vi "test_decodeTxGenConfig.vi"() -> ()   [LabVIEW 2020]
uses:
  Shared/hardware_channels_tx.ctl
  Shared/channel_settings_tx.ctl
  Shared/Frame Payload Parameters.ctl
  Shared/Encoding (Arinc664).ctl
  Shared/RawFrame_entry.ctl
  <instrlib>/AIM GmbH/_AIM 664/_controls/queue_header_generic.ctl
  <instrlib>/AIM GmbH/_AIM 664/AIM664LV.lvlib
panel:
  out "tx gen config":T1 {"channel settings"."Payload Parameter Array"."Parameters"."encoding" items=["BNR", "BCD", "Discrete"]}
  out "last mod":timestamp
  out "error out":errorcluster
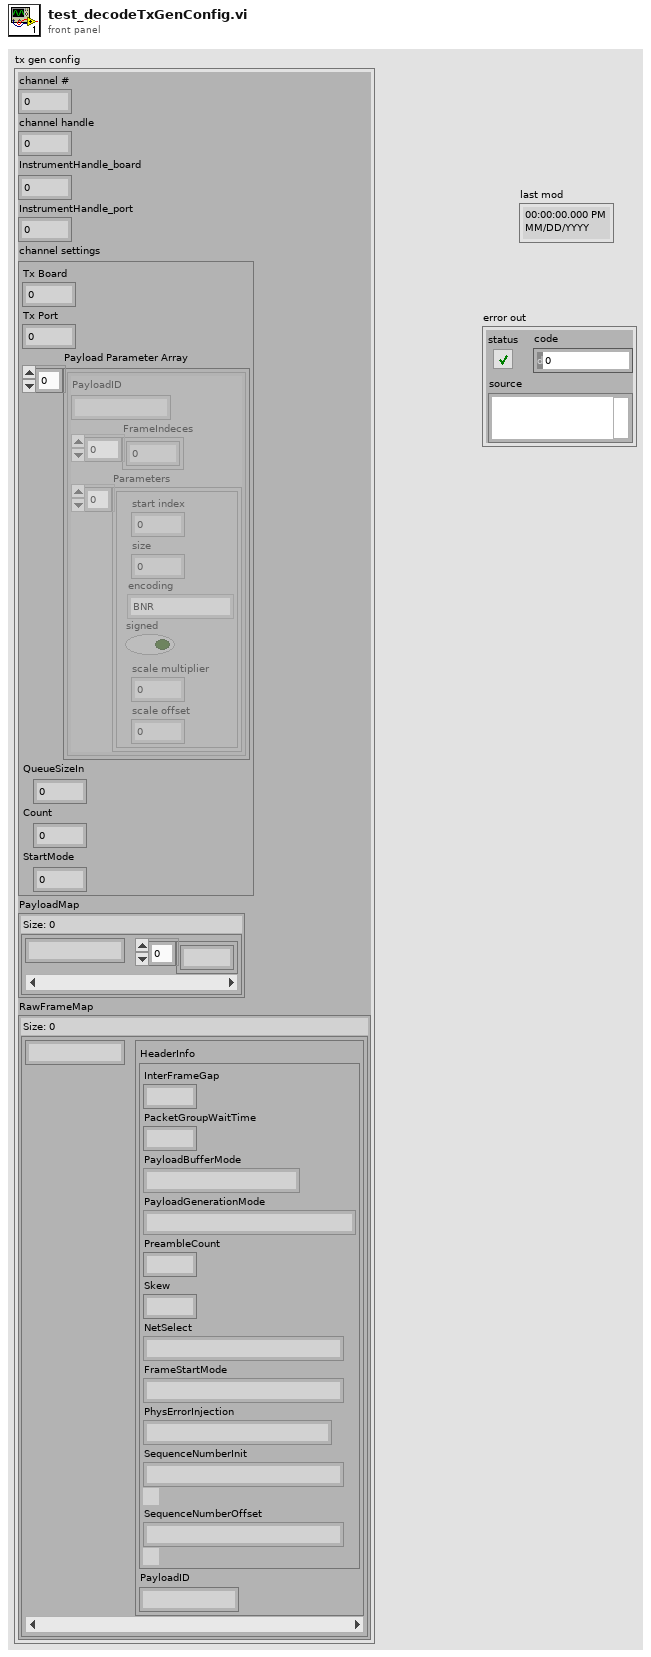
[diagram p1: front panel]
types:
  T1 = typedef "hardware_channels_tx.ctl" = cluster{"channel #":u16, "channel handle":u64, "InstrumentHandle_board":u32, "InstrumentHandle_port":u32, "channel settings":T2, "PayloadMap":map{string, u8[]}, "RawFrameMap":map{string, T5}}
  T2 = typedef "channel_settings_tx.ctl" = cluster{"Tx Board":u32, "Tx Port":u32, "Payload Parameter Array":T3[], "QueueSizeIn":u32, "Count":u32, "StartMode":u32}
  T3 = typedef "Frame Payload Parameters.ctl" = cluster{"PayloadID":string, "FrameIndeces":u32[], "Parameters":cluster{"start index":i32, "size":i32, "encoding":T4, "signed":bool, "scale multiplier":dbl, "scale offset":dbl}[]}
  T4 = typedef "Encoding (Arinc664).ctl" = u16
  T5 = typedef "RawFrame_entry.ctl" = cluster{"HeaderInfo":T6, "PayloadID":string}
  T6 = typedef "AIM664LV.lvlib/queue_header_generic.ctl" = cluster{"InterFrameGap":u32, "PacketGroupWaitTime":u32, "PayloadBufferMode":u8, "PayloadGenerationMode":u8, "PreambleCount":u8, "Skew":u32, "NetSelect":u8, "FrameStartMode":u8, "PhysErrorInjection":u32, "SequenceNumberInit":u16, "SequenceNumberOffset":u16}
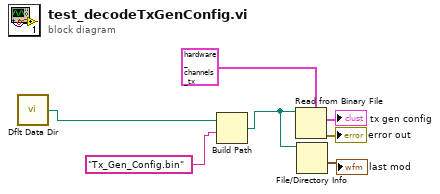
[diagram p0: block diagram]
diagram:
  n1 = call <vilib>:"Dflt Data Dir.vi"() -> ("App:Default Data Directory"=w7:path)
  n2 = Build Path(base path=w7, name or relative path="Tx_Gen_Config.bin" ("format string")) -> (appended path=w5:path)
  n3 = Read from Binary File(5:T1 {"channel #"=0, "channel handle"=0, "InstrumentHandle_board"=0, "InstrumentHandle_port"=0, "channel settings"={"Tx Board"=0, "Tx Port"=0, "Payload Parameter Array"=[], "QueueSizeIn"=0, "Count"=0, "StartMode"=0}, "PayloadMap"={}, "RawFrameMap"={}} ("Tx cluster out"), 11:w5) -> (0:→"error out":errorcluster, 2:→"tx gen config":T1)  [unwired: 4 in, 2 out]
  n4 = File/Directory Info(path=w5) -> (last mod=→"last mod":timestamp)  [unwired: 1 in, 6 out]
